vi "2-2.vi"() -> ()   [LabVIEW 2022 SP3, in "AoC22.lvlib"]
uses:
  AoC22.lvlib
  RPS Turn.ctl
  RPS Play.ctl
  RPS Result.ctl
  <vilib>/IlluminatedG/lv-stream/Stream.lvlib
panel:
  out "Score":i32
  out "Array":T1[](array[typedef])
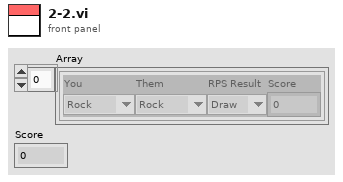
[diagram p1: front panel]
types:
  T1 = typedef "AoC22.lvlib/RPS Turn.ctl" = cluster{"You":T2, "Them":T2, "RPS Result":T3, "Score":i32}
  T2 = typedef "AoC22.lvlib/RPS Play.ctl" = enum16{"Rock", "Paper", "Scissors"}
  T3 = typedef "AoC22.lvlib/RPS Result.ctl" = enum16{"Draw", "Win", "Lose"}
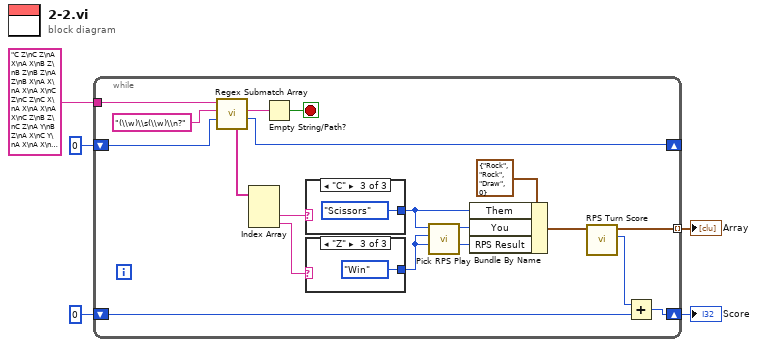
[diagram p0: block diagram]
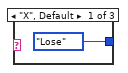
[diagram p2: hidden frame]
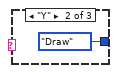
[diagram p3: hidden frame]
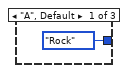
[diagram p4: hidden frame]
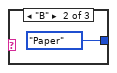
[diagram p5: hidden frame]
diagram:
  n1 = while {
    tunnel: "C Z\nC Z\nA X\nA X\nB Z\nB Z\nB Z\nA Z\nB X\nA X\nA X\nA X\nC Z\nC Z\nC X\nA X\nA X\nA X\nC Z\nB Z\nC Z\nA Y\nB Z\nA X\nC Y\nA X\nA X\nC Y\nC Z\nA Y\nB Z\nA X\nC Y\nB Z\nB Z\nB Z\nA X\nC X\nC X\nB Z\nA X\nC Z\nA X\nB Z\nA Y\nC X\nA X\nC Z\nC Z\nB Z\nC Y\nC X\nC X\nC X\nC X\nA Y\nC Y\nC Z\nC Y\nA X\nC Y\nA X\nB Z\nA Y\nC X\nA X\nB Y\nA X\nC X\nC X\nC Z\nA X\nC X\nA X\nC X\nB Z\nA Z\nB Y\nB Z\nB Z\nA X\nC Y\nB X\nA X\nA X\nB Z\nA X\nC X\nC Z\nC Z\nA X\nC Z\nC Z\nC Z\nC X\nC Z\nA X\nB Z\nB Y\nC Z\nB Z\nB Z\nA X\nB Z\nC Y\nC Z\nA X\nA Y\nC Z\nA X\nB Y\nC Y\nC Z\nA X\nC Y\nC X\nA X\nC X\nA X\nC Z\nA X\nC Y\nA Y\nC Z\nC X\nC Y\nC Y\nA Y\nA Y\nC Y\nC Y\nA Y\nA X\nC Z\nC Z\nC X\nC X\nC Z\nA Y\nC Z\nC Z\nA Y\nA Y\nB Z\nA X\nB Z\nC Y\nB Z\nC Z\nC Y\nC Y\nB Y\nC X\nA X\nA X\nA X\nA Y\nA X\nC Z\nC Z\nC Z\nA X\nB Z\nA X\nB Z\nC Y\nC Z\nA Y\nC Y\nA X\nA X\nC Z\nB X\nC Z\nC Z\nB Z\nB Z\nB Z\nC Z\nC X\nC Z\nA X\nB Z\nC Z\nC X\nA X\nA Y\nB Y\nA X\nB Z\nA X\nC Z\nC Z\nC X\nB Z\nC Z\nC Z\nC X\nA X\nA X\nB Y\nC Y\nC Z\nB Y\nA X\nB Z\nA X\nB X\nB Z\nC X\nC X\nC Y\nC X\nB Y\nB Z\nC X\nA Y\nC X\nC Y\nA X\nC Z\nC Z\nC X\nB Z\nA Y\nB Z\nA Y\nB X\nA X\nC Z\nB Z\nC X\nC X\nC X\nA X\nC X\nB Z\nC Z\nB Y\nB Z\nA X\nA X\nC Z\nB Z\nA X\nA Z\nC Y\nB Z\nC X\nC Z\nA Y\nC X\nA X\nA X\nA Y\nB Z\nA X\nB Z\nA Y\nB X\nC X\nC Y\nA X\nC Z\nB X\nC Z\nC X\nC X\nC Z\nA X\nB Z\nC Z\nC X\nC Z\nB Y\nA X\nC X\nC Y\nA X\nC Z\nA X\nB Z\nC X\nC X\nB Z\nC Z\nC Z\nC Y\nA X\nC Z\nC X\nA X\nC Y\nC Z\nC Z\nC Y\nB Y\nB Z\nA X\nB Y\nC X\nA X\nA X\nC Y\nC Z\nB Z\nC X\nC X\nB Z\nC Z\nA X\nA Y\nA X\nC Y\nA Y\nB Y\nA X\nA X\nC X\nC X\nB Z\nA Y\nB Z\nC Z\nA X\nA Y\nA X\nC X\nA X\nC Z\nB Y\nC Z\nA X\nB Z\nC Z\nC Z\nA X\nA X\nB Z\nB Z\nB Z\nA X\nC X\nA X\nA X\nC Y\nC Y\nC X\nC X\nA X\nA Y\nB Y\nC Z\nC Z\nB Y\nC X\nC Z\nA Y\nC X\nC Z\nC X\nB Z\nC Y\nC Z\nC X\nC Y\nC Z\nB Z\nC Z\nB Z\nA X\nB Y\nB Y\nC Z\nB Z\nC X\nC Z\nC Z\nC Z\nB Y\nB Z\nC Z\nB Y\nA X\nA X\nC X\nA X\nC X\nA X\nB Z\nA X\nA X\nA X\nC Z\nA Y\nA X\nC Z\nC X\nA X\nC X\nA X\nB Z\nC Z\nC Z\nC Z\nA X\nA X\nC Z\nA X\nB Z\nC X\nC Z\nC Y\nB Z\nA X\nB Z\nA X\nA Z\nB Y\nB Z\nB Z\nB Z\nA Y\nC Z\nA X\nB Y\nC X\nB X\nB Z\nC X\nB Y\nC Z\nA X\nC X\nB Z\nA X\nB Z\nA X\nA X\nB Y\nC Y\nC X\nC X\nC Z\nA X\nC Z\nA X\nB Y\nC X\nC Y\nB Y\nB Y\nA Y\nC X\nA Y\nC Z\nC Y\nA X\nC Z\nC Z\nB Z\nA X\nA X\nA X\nA X\nB Z\nC Z\nC X\nC X\nC Z\nA X\nB Z\nB Y\nC Y\nA Y\nC X\nB Z\nA Y\nB Z\nC Z\nB Z\nC X\nA X\nB Z\nA X\nA Y\nC Y\nB Z\nB Z\nC X\nC Z\nC Z\nC Z\nA X\nB Z\nA Y\nA X\nC Y\nA Y\nB Z\nA Y\nC Z\nA Y\nA Y\nC X\nA X\nB Z\nA Y\nB Z\nC X\nA X\nB Y\nB Z\nC Z\nC Z\nB Z\nA X\nA X\nB Y\nC Z\nC Y\nB Z\nC Z\nA Y\nA X\nC X\nC Z\nA X\nA X\nA Z\nC X\nC X\nB X\nB Z\nA Y\nC X\nA Y\nC X\nC Z\nA Y\nB Z\nA X\nB X\nA Y\nC X\nC Y\nA Y\nC X\nB Y\nC Y\nA X\nB Z\nA X\nC Z\nA X\nA X\nC Z\nC Z\nB X\nC X\nA Y\nB Z\nC Z\nA X\nA X\nC Z\nC Y\nA X\nC X\nC Z\nC Y\nC X\nC Y\nC X\nC Z\nC Z\nB Z\nA X\nA Y\nB Z\nA X\nB Z\nC X\nB Y\nA X\nA X\nA X\nA X\nB Z\nC Z\nB Z\nB Y\nC Z\nC X\nC Z\nC X\nB Z\nC Z\nA X\nC Z\nC Z\nA Y\nC X\nA X\nB Z\nA X\nB Z\nB Y\nA X\nA X\nA X\nA Y\nC Z\nA X\nB Y\nA Y\nB Y\nC Y\nA X\nA X\nC Y\nA X\nC Z\nB Z\nC X\nC Z\nA X\nB Z\nC Z\nB Z\nB Z\nB Z\nC X\nC Z\nA X\nA Y\nC X\nC Z\nB Z\nB Y\nC Z\nB Y\nB Z\nC Z\nA Y\nB Z\nC X\nC Y\nA X\nB Y\nA X\nC Z\nC X\nC Z\nA X\nC X\nB Z\nB X\nC Z\nB Z\nA Y\nA X\nA Y\nC Z\nC Y\nA X\nB X\nA Z\nC Y\nC X\nC Y\nC X\nC Y\nB Z\nC X\nB Y\nC Z\nC Y\nB Z\nA Y\nB Y\nC Z\nC X\nB Z\nA Y\nC Z\nC Z\nC Z\nC Y\nC X\nC X\nB Y\nC Z\nA Y\nC Z\nC X\nB Y\nC X\nB Z\nB Z\nB Z\nB Z\nC Y\nC Z\nC X\nB X\nC Z\nC Z\nC Z\nC X\nB Y\nB Z\nC X\nA X\nC Y\nB X\nC X\nC X\nC Z\nA X\nA X\nB Z\nB Z\nA X\nC Z\nA X\nA Y\nC X\nB X\nC Y\nC Y\nA X\nA X\nC Z\nC Z\nB Y\nB Y\nB Z\nC X\nA X\nA Z\nC Z\nB Y\nC Y\nC X\nC Y\nB Z\nC X\nA X\nA X\nC Z\nC Y\nB X\nC Z\nB Z\nA X\nC X\nA Y\nC Y\nC Z\nB Z\nC Z\nA X\nC Y\nB Z\nC Y\nB X\nC Z\nC Z\nA X\nA X\nC X\nC Z\nC X\nC Y\nC Z\nA Y\nC X\nC Z\nB Y\nB Y\nC Z\nA X\nC Y\nA X\nC X\nC X\nB Y\nC Z\nC Z\nA X\nA Y\nC Z\nB Z\nC Y\nA X\nA X\nC Z\nC Z\nA X\nC Z\nC Z\nB Z\nB Z\nA X\nA Y\nA X\nC Z\nC X\nA X\nB X\nC Z\nC Z\nB Y\nA X\nB Z\nC X\nC Z\nC Z\nC Z\nC X\nA Y\nA X\nA Y\nA X\nA Y\nC Z\nC Z\nB Z\nB Y\nA X\nB Z\nC Z\nC X\nC Y\nC Z\nA X\nC Y\nB Y\nB Z\nC Z\nB Y\nC X\nC Z\nB Y\nB Z\nB Y\nC X\nC Z\nC X\nC Z\nB Y\nB Z\nC X\nA X\nA Y\nB Z\nB Y\nA X\nA X\nC Z\nA X\nA X\nC X\nA X\nC Z\nC X\nA X\nB X\nA Y\nC X\nA X\nC Y\nA X\nC Z\nA X\nA X\nC Z\nA X\nA X\nC Z\nA X\nB Y\nB Z\nA X\nC X\nA X\nC X\nB Z\nC Y\nA Y\nC Z\nB Z\nA X\nC X\nA X\nB Y\nC X\nB Y\nB Z\nA X\nB Z\nC X\nB Z\nA X\nA X\nC X\nA X\nC X\nA Y\nC Z\nA X\nB Y\nB Z\nC Z\nC Z\nA X\nC Y\nB Z\nC X\nB Z\nB Z\nC Z\nA X\nC X\nC X\nA Y\nA X\nC Z\nB Z\nA X\nB X\nA X\nB Z\nB Z\nC Z\nB Y\nC Z\nA X\nC Z\nC Z\nC Z\nC X\nA X\nA X\nC Y\nB Y\nC Z\nB Y\nA X\nB Z\nA Y\nC Y\nB Y\nC Z\nC X\nC X\nA X\nB Y\nA X\nA X\nC Z\nC X\nC Y\nA X\nA X\nA X\nC X\nB Z\nB Y\nA X\nB Y\nC X\nC Z\nB Z\nA X\nC X\nC Z\nB Y\nA X\nC Z\nB Z\nB Z\nA X\nB Y\nA X\nB Y\nC Z\nC Z\nB Z\nC Z\nC Y\nA X\nB Z\nC Z\nA Y\nC Z\nB Z\nB Z\nC Z\nB Y\nC Z\nC Z\nB Z\nA Y\nC X\nC Y\nB Z\nC X\nC Z\nA X\nA X\nC Y\nA Z\nC Z\nC X\nB Z\nB Z\nC Y\nA X\nA Y\nC Z\nA X\nA X\nB Z\nA X\nC X\nC X\nB X\nB X\nA Z\nB Y\nA X\nA Y\nC Z\nA X\nA X\nB Z\nB Z\nC Y\nA X\nC Y\nC Z\nA Y\nC Y\nB X\nC X\nA X\nB Z\nA X\nA X\nA X\nA X\nA X\nB X\nA X\nC Z\nB Z\nB Z\nB X\nA X\nC Z\nB Z\nC Z\nC Z\nC Y\nA X\nC Y\nC Y\nC Z\nA Y\nC Z\nA X\nC X\nC Z\nA X\nA Y\nC Z\nC X\nA X\nC X\nB Y\nC Z\nB Z\nA X\nC Y\nB Z\nB Y\nA X\nC Z\nA X\nB Z\nC Z\nC Y\nC Z\nA X\nA X\nB Z\nB Y\nA X\nC X\nC Y\nB X\nC Z\nA Y\nC X\nB Y\nB Z\nA Y\nC Y\nC Z\nC Z\nC X\nA X\nA X\nC X\nC X\nC Z\nC X\nC X\nB X\nB Z\nB Z\nC X\nC Z\nC X\nA X\nA X\nA X\nC Z\nC Y\nB Z\nC X\nC X\nA X\nC X\nC Y\nA X\nB Y\nA X\nC Z\nC Z\nB Z\nA X\nA X\nA X\nB Z\nC X\nA X\nB Y\nB Z\nC X\nB Y\nC X\nB Y\nC Z\nB X\nA X\nA X\nB Z\nA X\nA X\nA X\nB Z\nA X\nC Z\nC X\nC Z\nA X\nC Y\nC Y\nC Z\nC Z\nC Z\nA X\nC Z\nC X\nC Z\nC Z\nA X\nB Z\nC X\nC Y\nB X\nB Z\nB Z\nA X\nC Y\nB Y\nC Z\nB Z\nC Z\nC X\nA Z\nC Z\nB X\nC X\nC Z\nC Z\nC X\nC Z\nC Z\nA X\nB Z\nC Z\nC X\nA X\nB Z\nC Y\nC Y\nB Y\nC X\nA X\nA X\nC Z\nB Z\nC X\nC X\nC X\nB Y\nC Z\nB X\nC X\nC Z\nA X\nA X\nC Z\nC Z\nC X\nC X\nC Z\nA X\nC Z\nC X\nC Z\nC Z\nA X\nC Z\nA X\nA X\nA X\nB Z\nA X\nB Z\nC Z\nC Z\nA X\nC Z\nC Z\nB Z\nC Z\nA Y\nC X\nA X\nA X\nC X\nA X\nC X\nC X\nA Y\nB Y\nC Z\nB Z\nC X\nB Y\nC Y\nC X\nC Z\nA X\nC Y\nB Z\nB Y\nA X\nB Y\nB Y\nA X\nC X\nC X\nA X\nA Y\nC Y\nB Z\nA X\nB Z\nA Y\nB Y\nC Z\nC Z\nC Z\nA Y\nB Y\nB Y\nC Z\nB Z\nC Z\nA X\nC Y\nA X\nB Y\nB Z\nC X\nC Y\nA X\nB Z\nB Z\nA X\nB Z\nC Y\nA X\nC X\nC Z\nC Z\nA X\nC Y\nA X\nC X\nC X\nB Z\nB Y\nA X\nC Y\nB Z\nB Y\nA X\nC Z\nA X\nB Y\nA X\nA X\nA X\nC X\nA X\nC Z\nB Z\nC Z\nA X\nA X\nB Y\nC X\nC Y\nC Z\nA X\nC Z\nB Z\nA X\nB Z\nA X\nB Y\nB Z\nC Z\nC Z\nC Y\nC X\nA X\nC Z\nA Y\nA X\nB Z\nB Y\nA X\nC X\nC Z\nB Z\nA X\nC Z\nC X\nC Y\nA X\nA X\nC Z\nA X\nA X\nC X\nC X\nA X\nC X\nC Z\nA X\nA X\nC Y\nA Y\nB Z\nC X\nC X\nB Y\nB Z\nA X\nB Z\nC Z\nC Z\nA Y\nC Y\nC Z\nA X\nC Z\nA X\nC Y\nC X\nB X\nB Z\nA X\nA X\nB Z\nA X\nC X\nC X\nA Y\nA X\nA X\nC Y\nB Z\nA X\nB Y\nC X\nB Z\nC Y\nB Y\nA X\nC Z\nB Y\nB Z\nA X\nB Y\nC X\nC Z\nA X\nB Z\nA X\nC Y\nC Z\nA X\nA X\nC Y\nC Y\nC X\nA Y\nC Z\nB Z\nA X\nA Y\nC Z\nC Z\nC Z\nC Z\nB Y\nA Y\nA X\nA X\nC X\nA X\nB Y\nC Z\nB Z\nA Y\nC X\nC X\nA Y\nA X\nA X\nC X\nC Z\nC X\nA X\nA Y\nC X\nC Z\nC X\nA X\nA X\nC Z\nC X\nA X\nC X\nC Z\nA X\nA X\nC Z\nB Y\nA X\nC Z\nC Y\nC Z\nC Z\nB X\nB Z\nB X\nA X\nC Z\nB X\nC Z\nA X\nC Z\nA Y\nA Z\nB Z\nC X\nA X\nA X\nA X\nA X\nA X\nC Z\nA X\nB X\nA Y\nA X\nC X\nA X\nA Y\nA Y\nB Y\nC X\nA Y\nA X\nC Z\nC Z\nC Y\nB Z\nC X\nC Z\nA Y\nC X\nC Y\nC X\nA X\nB Y\nC Z\nC Z\nA X\nC Z\nB Z\nB Z\nC X\nC X\nA X\nB Y\nC X\nC X\nA X\nC Z\nB Y\nC Y\nC Z\nA X\nB Z\nC Z\nB Y\nC X\nA X\nB Y\nB Z\nA X\nC Y\nB Z\nC Z\nC X\nA X\nC X\nA X\nB Y\nC X\nA X\nC Y\nB Z\nB Z\nB Z\nC Y\nA X\nA X\nA Y\nC Z\nB X\nB Z\nA X\nA X\nC X\nA X\nC X\nA X\nC X\nA X\nA X\nA X\nA Y\nA Y\nB Y\nA X\nB Y\nA X\nB Y\nB Z\nB Y\nA Y\nC Z\nC Z\nC Z\nC Z\nA X\nC Z\nC X\nC Y\nC Z\nB Z\nB Z\nB Z\nC Y\nC Z\nB Z\nC X\nA Y\nA X\nC X\nC Y\nA Y\nB Y\nC X\nC X\nB Y\nC Z\nA X\nC X\nC X\nC X\nC X\nC X\nC X\nB Z\nC Y\nA X\nA X\nB Y\nB Z\nA X\nC X\nC Z\nA X\nB X\nB Z\nC Y\nB Z\nC Z\nC Y\nA X\nC Z\nB Y\nC X\nA X\nA Y\nA X\nC X\nA Y\nA Y\nC Z\nB Z\nC Z\nC X\nC Y\nB Y\nA X\nC X\nC Z\nB Y\nA X\nB X\nB Z\nC Z\nB Z\nB Z\nA X\nA Y\nA X\nA X\nB Z\nC Z\nA X\nA Y\nC Z\nC Z\nC Y\nA X\nB Z\nC X\nC X\nA Y\nA X\nC X\nC Y\nC Z\nC Y\nC X\nA X\nB Z\nC Y\nB Z\nC X\nA X\nA X\nC X\nC Z\nC Y\nC Y\nA X\nA Y\nC Z\nA Y\nB Y\nC Y\nA Y\nC Z\nB Y\nC X\nA X\nB Z\nC Z\nA X\nA X\nB Z\nC X\nB Z\nC Z\nC Z\nA Y\nA X\nC X\nA X\nB Z\nC X\nA X\nA X\nB Y\nA Z\nB Z\nC X\nC Z\nC X\nC Z\nC X\nA X\nC Z\nB Y\nC Y\nC Z\nA X\nC Z\nA X\nA Z\nA X\nA X\nC Z\nA X\nB Z\nC X\nB Z\nA X\nC X\nA X\nC X\nC Z\nB Z\nA Y\nC Y\nC Z\nC Z\nC X\nC Z\nA X\nA X\nB Y\nB Z\nC Y\nB Z\nA Y\nA X\nA X\nB Z\nB X\nA X\nB Y\nB Z\nC X\nA X\nA X\nC Z\nB Y\nC X\nB Y\nA Y\nA Z\nA X\nB Y\nC X\nC Z\nC Z\nC Y\nC Z\nA X\nB X\nC X\nA Y\nA X\nC Z\nC Y\nC X\nB Z\nA X\nC X\nC Z\nA X\nC Z\nA X\nC X\nC X\nA Y\nC Z\nA X\nC X\nC Z\nC Y\nA X\nA Y\nA Y\nC Z\nC X\nA X\nC Z\nA Y\nA Y\nA X\nB Z\nC Z\nB Y\nC Z\nB Y\nC X\nC Z\nB Y\nA X\nA X\nB Z\nA X\nC Z\nA X\nA X\nB Y\nA X\nB Z\nA Y\nA X\nA Y\nC Z\nB Z\nA X\nB X\nB Y\nB Z\nA X\nA Z\nB Y\nB Z\nC X\nB Z\nA X\nB Z\nC Z\nB Y\nC X\nA X\nA Y\nB Y\nA Y\nC X\nC X\nB Y\nA Y\nB Z\nC Z\nB Z\nA Y\nA X\nB Z\nB Z\nA Y\nC Z\nC Z\nB Z\nC X\nB Z\nB Y\nB Z\nB Z\nA X\nA X\nC X\nC Z\nB Z\nA X\nB Z\nC Y\nC Z\nA Z\nA X\nA X\nC Z\nA X\nC Z\nC Z\nC Z\nB Z\nA X\nA Y\nB X\nA X\nA X\nA X\nC Z\nB X\nB X\nA X\nC Z\nA X\nB X\nA X\nA X\nB Z\nA X\nC Z\nC Y\nA X\nB Z\nA X\nC Z\nB Z\nA X\nA X\nB Y\nB Y\nC Y\nA X\nB Z\nC Y\nA X\nC Z\nB Z\nA X\nC Z\nB Z\nC X\nB X\nB Z\nC Z\nA X\nB Z\nA X\nA X\nA X\nA X\nC Z\nB Z\nB Y\nC Z\nA X\nC Z\nA X\nC X\nC X\nA X\nB Y\nC X\nB Z\nA Y\nC Y\nB Z\nC Y\nC X\nA X\nB Z\nC X\nB Y\nA X\nA Y\nB Y\nB Y\nA X\nC X\nC Z\nB Z\nA Y\nA X\nB Y\nC X\nB Z\nB X\nC Y\nB X\nC X\nB Y\nC X\nA X\nC Z\nB Z\nB Y\nB Y\nA X\nA X\nA Z\nB Z\nB Z\nC X\nC Y\nA Y\nC Z\nC X\nA X\nC Z\nC X\nB Z\nA Y\nB Z\nC Z\nB Z\nB Z\nC X\nB Z\nC X\nC X\nB Z\nA X\nB Y\nB Z\nA X\nC X\nA X\nC Y\nA X\nC X\nB X\nC Z\nC Y\nC Z\nB Z\nC X\nA X\nA X\nA Y\nC Z\nC Y\nA Y\nC Z\nB Z\nC Z\nC Y\nA X\nA X\nC X\nC Z\nC Z\nA Z\nC Z\nA X\nB Z\nC X\nC Z\nA X\nB Z\nC X\nA X\nA Y\nB Y\nC X\nA X\nA X\nC X\nC Y\nB Z\nC X\nA X\nC X\nB Z\nB Y\nA Y\nC Z\nA X\nC Z\nC Z\nA X\nC Y\nB Z\nA Y\nB Y\nB Y\nA X\nA X\nC X\nC X\nB Y\nC Z\nC Z\nC Z\nC X\nC Y\nC Z\nB Z\nC Z\nA Y\nC Z\nA X\nB Z\nB Y\nB Z\nA X\nA X\nA X\nA X\nC X\nC Z\nB Z\nC X\nB Z\nC Z\nA X\nC X\nC Z\nB Y\nA X\nC X\nA X\nB Z\nB Z\nA X\nA X\nB Y\nC Y\nC Y\nC X\nA X\nB Z\nC Y\nB Z\nA Y\nB Y\nB Y\nA X\nB Z\nA X\nC X\nC Z\nA X\nB Z\nA Y\nC Y\nB Z\nC Z\nC Y\nA X\nC Y\nA X\nC X\nB Z\nC X\nA X\nC Z\nA X\nB Y\nB Z\nC X\nC Y\nB X\nA X\nB Z\nA X\nB Y\nC X\nC X\nC Y\nC Y\nC X\nB Y\nC Z\nC X\nB Z\nB Y\nC X\nA Y\nC Z\nC Z\nC X\nB X\nB Y\nA X\nA X\nC Z\nC X\nC Y\nA X\nC Y\nA Y\nC Z\nC X\nA X\nC Z\nC X\nA X\nB X\nC X\nC X\nC X\nB Y\nB Z\nC X\nC Z\nA Y\nB Y\nC X\nC X\nA X\nB Z\nC Z\nA X\nC Y\nC Z\nA Y\nB Z\nC X\nC Z\nA X\nC Z\nB Z\nB Y\nB Z\nA X\nC X\nA Y\nC X\nC Z\nB Y\nC Y\nC Z\nC Z\nA X\nA X\nA X\nC Z\nB Y\nC Z\nA X\nA X\nB Z\nB Y\nB Z\nC Z\nB Z\nA Y\nC Y\nC Z\nB Y\nA X\nA X\nC Z\nB Y\nC Z\nA X\nC X\nB Y\nA Y\nB Z\nA X\nA X\nA X\nB Y\nA X\nC Z\nB Y\nC Z\nB Y\nC Z\nC X\nC Y\nC X\nA X\nA X\nA X\nC Z\nC X\nC X\nB Y\nA Y\nB Z\nB X\nC Z\nB Y\nA X\nC Y\nB Z\nC X\nA X\nA X\nA X\nA X\nC X\nB Y\nA X\nA X\nB Y\nA X\nB Z\nC Z\nA X\nA X\nA X\nA X\nB Z\nA X\nC Z\nC X\nC Y\nB Z\nC Z\nA X\nC Y\nC Z\nA X\nA X\nC X\nB Z\nC X\nB Z\nC Z\nA X\nA X\nA Y\nB Y\nC Z\nB Y\nA X\nC X\nC Z\nC Z\nC X\nA X\nA X\nC Z\nA X\nA Y\nA X\nA X\nC Z\nC X\nC X\nC Z\nC X\nA X\nC Z\nC Z\nB Z\nA Y\nA Y\nB Y\nA X\nA X\nC X\nC X\nA X\nA X\nC X\nC X\nB Y\nC Z\nA X\nB Y\nA X\nA X\nA X\nC X\nC Y\nB Z\nB Y\nB Z\nC Z\nC Z\nC X\nC Z\nA X\nB Z\nA Y\nC Z\nB Z\nA X\nC Y\nB Z\nC Z\nC Y\nA X\nB Y\nC Z\nA X\nA X\nA X\nC Z\nC Z\nC X\nA Y\nC X\nB Z\nB Y\nA X\nC X\nC X\nA Y\nA Y\nA X\nB X\nB Z\nB Y\nB Y\nA X\nC Y\nA X\nC Z\nC X\nC X\nC Z\nB Z\nB Z\nC Y\nC X\nB Z\nC Z\nA Y\nC Y\nA X\nB Z\nA X\nC Y\nB Z\nB Y\nC Z\nA X\nA X\nC Z\nB Z\nB Z\nC Z\nC Y\nC Z\nC Z\nC X\nA Y\nA Y\nB Z\nC Z\nB Y\nC X\nC X\nA Z\nC Z\nA X\nA X\nC X\nA Y\nC X\nA X\nA X\nA X\nC Y\nA X\nB Y\nA X\nB Y\nA X\nA X\nA Y\nC X\nC Z\nA X\nC X\nB Y\nB Z\nB Z\nA Y\nC Z\nC X\nC X\nB Z\nB Z\nC X\nB Y\nA X\nB Y\nA X\nA X\nC Y\nB X\nC X\nA Z\nA Z\nA X\nC Z\nC Y\nC Z\nC Y" -> [w23]
    shift-right: [w20] -> _
    shift-left: 0 -> [w21]
    tunnel: [w12] -> w3 mode=indexing
    shift-right: [w9] -> w1
    shift-left: 0 -> [w11]
    stop <- w18 stop-if-true
    n2 = call <vilib>:"Regex Submatch Array.vi"("offset (0)"=w21, "regular expression"="(\\w)\\s(\\w)\\n?", "string"=w23) -> ("offset past match"=w20:i32, "after match"=w19:string, "matches"=w17:string[])  [unwired: 4 in, 2 out]
    n3 = Index Array(array=w17) -> (element #2=w16:string, element #3=w15:string)  [unwired: 3 in, 1 out]
    n4 = Empty String/Path?(string/path=w19) -> (empty?=w18:bool)
    n5 = case shown="\"C\"" w16 {
      tunnel: [RPS_Play."Rock" ("RPS Play") RPS_Play."Paper" ("RPS Play") RPS_Play."Scissors" ("RPS Play")] -> w8
      frame "A", Default {
      }
      frame "B" {
      }
      frame "C" {
      }
    }
    n6 = case shown="\"Z\"" w15 {
      tunnel: [RPS_Result."Lose" ("RPS Result") RPS_Result."Draw" ("RPS Result") RPS_Result."Win" ("RPS Result")] -> w7
      frame "X", Default {
      }
      frame "Y" {
      }
      frame "Z" {
      }
    }
    n7 = call "Pick RPS Play.vi"("Result"=w7, "Them"=w8) -> ("You"=w6:T2)  [unwired: 9 in]
    n8 = Bundle By Name(cluster=T1 {"You"=enum."Rock", "Them"=enum."Rock", "RPS Result"=enum."Draw", "Score"=0} ("RPS Turn"), "Them"=w8, "You"=w6, "RPS Result"=w7) -> (w13:T1)
    n9 = call "RPS Turn Score.vi"("RPS Turn In"=w13) -> ("Score"=w10:i32, "RPS Turn"=w12:T1)  [unwired: 9 in]
    n10 = Add(x=w10, y=w11) -> (x+y=w9:i32)
  }
  "Array" <- w3
  "Score" <- w1
